vi "认识while循环2.vi"() -> ()   [LabVIEW 2018]
panel:
  out "字符串":string="从数组中循环读取元素\n需要注意i值和数组大小的比较"
  in  "停止":bool
  out "当前循环i":i32
  out "当前实时数据":dbl
  in  "数组":dbl[](array[numeric])
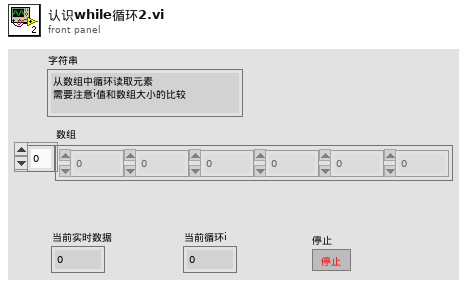
[diagram p1: front panel]
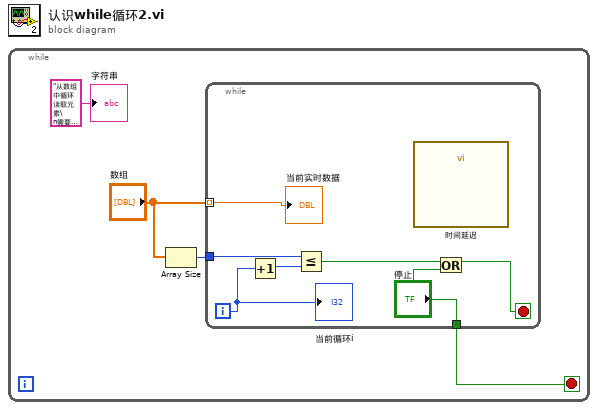
[diagram p0: block diagram]
diagram:
  n1 = while {
    stop <- w1 stop-if-true
    n2 = Array Size(array="数组") -> (size(s)=w3:i32)
    n3 = while {
      tunnel: "数组" -> [w11] mode=indexing
      tunnel: w3 -> [w8]
      tunnel: ["停止"] -> w1
      i -> [w10]
      stop <- w6 stop-if-true
      n4 = Increment(x=w10) -> (x+1=w7:i32)
      n5 = Less Or Equal?(x=w8, y=w7) -> (x <= y?=w9:bool)
      n6 = call "时间延迟"() -> ()  [unwired: 11 in, 1 out]
      n7 = Or(x=w9, y="停止") -> (x .or. y?=w6:bool)
      "当前实时数据" <- w11
      "当前循环i" <- w10
    }
    "字符串" <- "从数组中循环读取元素\n需要注意i值和数组大小的比较"
  }
